vi "Joy to XBox.vi"(6 "Joystick Deadband":dbl, 10 "JoystickDevRef":T1) -> (2 "Xbox One Controller":T3 {"Right Joystick"."Right" min=-1.0 max=1.0 step=0.1 scale=-1.0..1.0; "Right Joystick"."Forward" min=-1.0 max=1.0 step=0.1 scale=-1.0..1.0; "Left Joystick"."Right" min=-1.0 max=1.0 step=0.1 scale=-1.0..1.0; "Left Joystick"."Forward" min=-1.0 max=1.0 step=0.1 scale=-1.0..1.0})   [LabVIEW 2014, in "Xbox One Controller.lvlib"]
uses:
  Xbox One Controller.lvlib
  Xbox One Controller State.ctl
  Joystick.ctl
  <vilib>/Rock Robotics/WPI/Joystick/WPI_JoystickDevRef.ctl
  <vilib>/Rock Robotics/WPI/Joystick/WPI_JoystickDeviceEnum.ctl
panel:
  out "Buttons":bool[](array[boolean])
  out "POVs":i16[](array[numeric])
  out "Axes":dbl[](array[numeric])
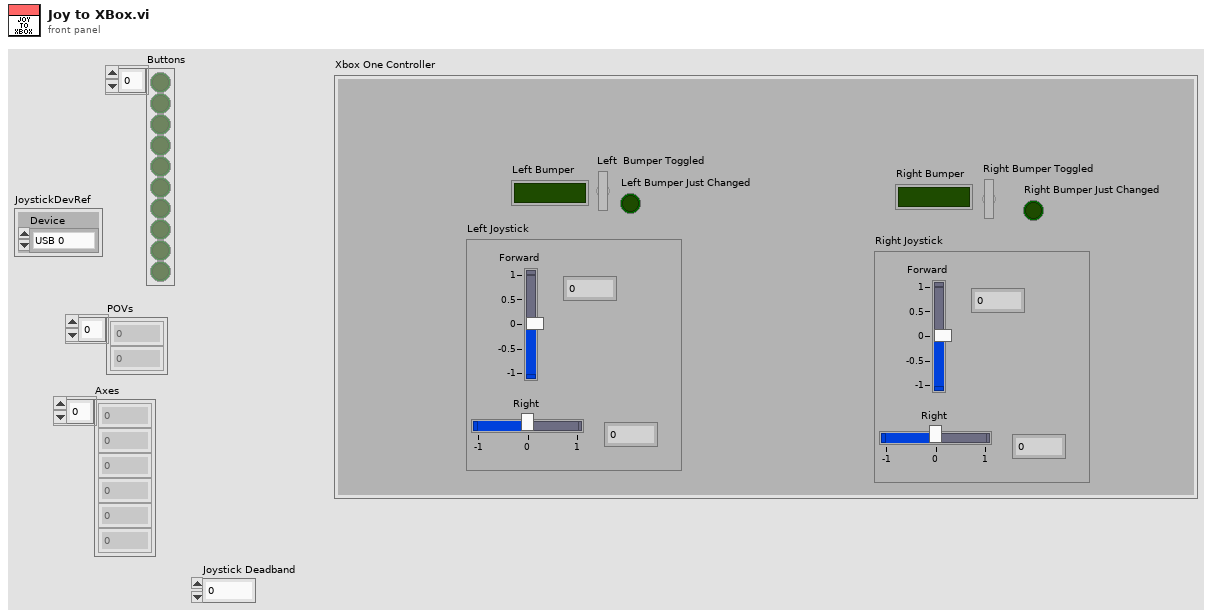
[diagram p1: front panel]
types:
  T1 = typedef "WPI_JoystickDevRef.ctl" = cluster{"Device":T2}
  T2 = typedef "WPI_JoystickDeviceEnum.ctl" = enum16{"USB 0", "USB 1", "USB 2", "USB 3", "USB 4", "USB 5"}
  T3 = typedef "Xbox One Controller.lvlib/Xbox One Controller State.ctl" = cluster{"Left Joystick":T4, "Right Joystick":T4, "Right Bumper":bool, "Left Bumper":bool, "Left  Bumper Toggled":bool, "Right Bumper Toggled":bool, "Left Bumper Just Changed":bool, "Right Bumper Just Changed":bool}
  T4 = typedef "Xbox One Controller.lvlib/Joystick.ctl" = cluster{"Forward":dbl, "Right":dbl}
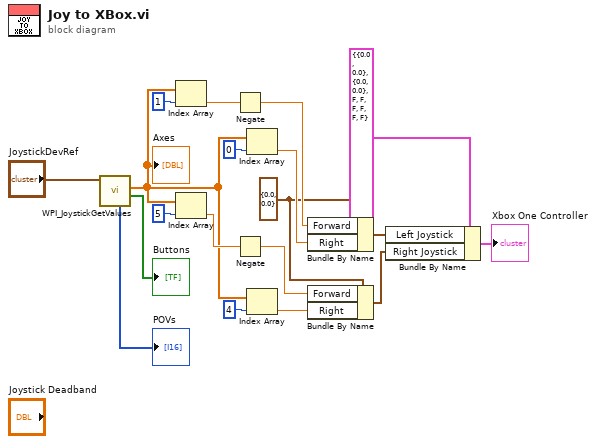
[diagram p0: block diagram]
diagram:
  w8 = T4 {"Forward"=0.0, "Right"=0.0} ("Left Joystick")
  n1 = call <vilib>:"WPI_JoystickGetValues.vi"("JoystickDevRef"="JoystickDevRef") -> ("Buttons"=→"Buttons":bool[], "Axes"=w3:dbl[], "POVs"=→"POVs":i16[])  [unwired: 6 in, 2 out]
  "Axes" <- w3
  n2 = Index Array(array=w3, index=1) -> (element=w12:dbl)
  n3 = Index Array(array=w3, index=5) -> (element=w6:dbl)
  n4 = Negate(x=w12) -> (-x=w11:dbl)
  n5 = Negate(x=w6) -> (-x=w5:dbl)
  n6 = Index Array(array=w3, index=0) -> (element=w9:dbl)
  n7 = Index Array(array=w3, index=4) -> (element=w2:dbl)
  n8 = Bundle By Name(cluster=w8, "Forward"=w11, "Right"=w9) -> (w14:T4)
  n9 = Bundle By Name(cluster=w8, "Forward"=w5, "Right"=w2) -> (w1:T4)
  n10 = Bundle By Name(cluster=T3 {"Left Joystick"={"Forward"=0.0, "Right"=0.0}, "Right Joystick"={"Forward"=0.0, "Right"=0.0}, "Right Bumper"=FALSE, "Left Bumper"=FALSE, "Left  Bumper Toggled"=FALSE, "Right Bumper Toggled"=FALSE, "Left Bumper Just Changed"=FALSE, "Right Bumper Just Changed"=FALSE} ("Xbox One Controller"), "Left Joystick"=w14, "Right Joystick"=w1) -> (→"Xbox One Controller":T3)
